vi "Corect settings.vi"(0 "NewVal":T1 {"delta level" min=0.0 max=10.0 step=1.0}, 9 "OldVal":T1 {"delta level" min=0.0 max=10.0 step=1.0}) -> (4 "Setting PMG":T1 {"delta level" min=0.0 max=10.0 step=1.0})   [LabVIEW 2019, in "GUI PumpMotorGroup.lvclass"]
uses:
  GUI PumpMotorGroup.lvclass
  TypeDef/GUI Setting PMG.ctl
panel:
  # "НС Охлаждения и отчистки (М24)"
  # "НС Подачи масла (М21)"
  # "НС Перекачки масла (М12)"
  # "НС Охлаждения и отчистки (М24)"
  # "НС Подачи масла (М21)"
  # "НС Перекачки масла (М12)"
  # "НС Охлаждения и отчистки (М24)"
  # "НС Подачи масла (М21)"
  # "НС Перекачки масла (М12)"
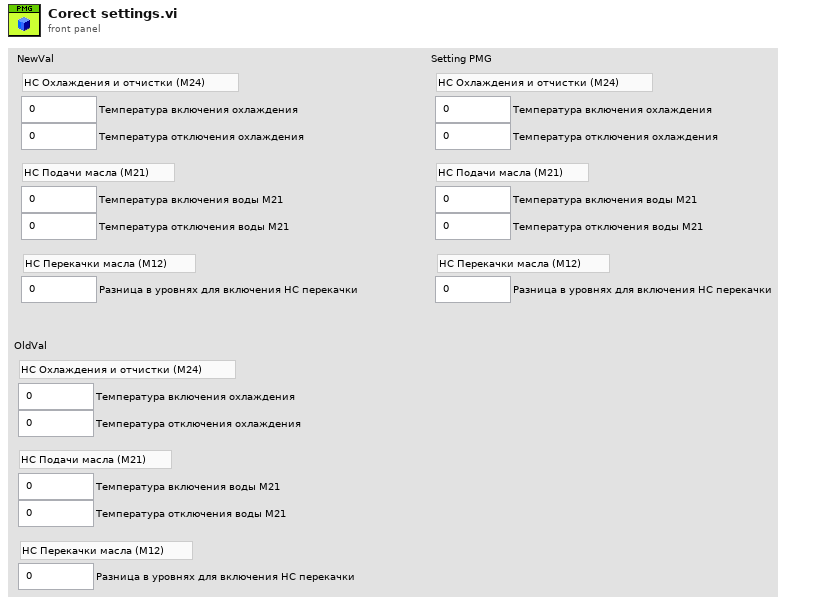
[diagram p1: front panel]
types:
  T1 = typedef "GUI Setting PMG.ctl" = cluster{"Temp Turn ON M24":dbl, "Temp Turn OFF M24":dbl, "Temp Open Water M21":dbl, "Temp Close Water M21":dbl, "delta level":dbl}
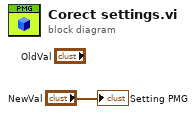
[diagram p0: block diagram]
diagram:
  "Setting PMG" <- "NewVal"
